vi "Planta lazo abierto.vi"() -> ()   [LabVIEW 2022 SP3]
uses:
  <vilib>/MakerHub/LINX/Public/Peripherals/PWM/PWM Set Duty Cycle 1 Chan.vi
  <vilib>/MakerHub/LINX/Public/Utilities/Open Serial.vi
  <vilib>/MakerHub/LINX/Public/Peripherals/PWM/PWM Set Duty Cycle N Chans.vi
  <vilib>/MakerHub/LINX/LMH-LINX.lvlib
panel:
  in  "Stop Button":bool
  out "Waveform Chart":cluster{dbl, dbl}(graph)
  in  "Set Point":dbl(slide) scale=0.0..100.0
  out "RPM":dbl(knob) scale=0.0..1500.0
  in  "Serial Port":refnum<visa-resource-name>="N/A"
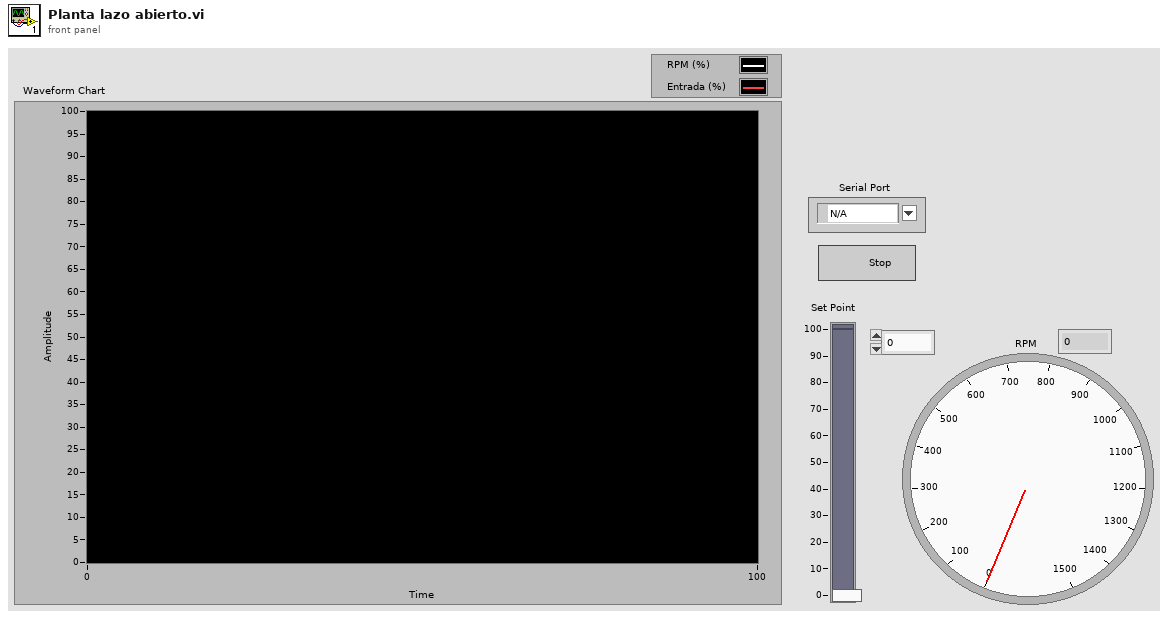
[diagram p1: front panel]
types:
  T1 = typedef "LMH-LINX.lvlib/LINX Ref.ctl" = cluster{"IO":T2, "Interface":T3, "LINX Device Config":T4}
  T2 = typedef "LMH-LINX.lvlib/Platform.ctl" = enum16{"Remote", "Local"}
  T3 = typedef "LMH-LINX.lvlib/Interface.ctl" = enum16{"Serial", "TCP"}
  T4 = typedef "LMH-LINX.lvlib/Device.lvlib/LINX Device Config.ctl" = cluster{"Interface":T3, "COM Port":refnum<visa-resource-name>, "TCP Configuration":T5, "Device Family":u8, "Device ID":u8, "Device Name":string, "TCP Ref":refnum<k5>, "Channels":T6}
  T5 = typedef "LMH-LINX.lvlib/Device.lvlib/TCP Config.ctl" = cluster{"IP Address":string, "Port":u16}
  T6 = typedef "LMH-LINX.lvlib/Channels.ctl" = cluster{"DI":u8[], "DO":u8[], "AI":u8[], "AO":u8[], "PWM":u8[], "QE":u8[], "UART":u8[], "I2C 2":u8[], "SPI":u8[], "CAN":u8[], "Servo":u8[], "AI Ref (V)":dbl, "AI Resolution (Bits)":u8, "AO Ref (V)":dbl, "AO Resolution (Bits)":u8}
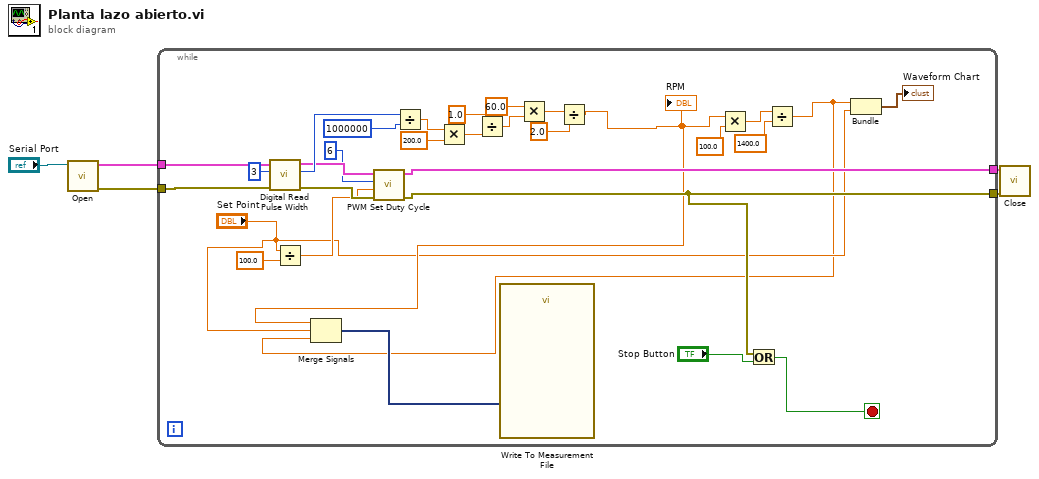
[diagram p0: block diagram]
diagram:
  n1 = call-poly <vilib>:"Open.vi"("Serial Port"="Serial Port") -> ("Error Out"=w3:errorcluster, "LINX Resource"=w4:T1)  [unwired: 8 in, 1 out]
  n2 = while {
    tunnel: w4 -> [w35]
    tunnel: w3 -> [w33]
    tunnel: [w24] -> w2
    tunnel: [w15] -> w1
    stop <- w17 stop-if-true
    n3 = call <vilib>:"Digital Read Pulse Width.vi"("Error In"=w33, "DI Channel"=u8 3, "LINX Resource"=w35) -> ("Error Out"=w23:errorcluster, "Pulse Width (uS)"=w32:u32, "LINX Resource"=w25:T1)  [unwired: 6 in]
    n4 = Divide(x="Set Point", y=100.0) -> (x/y=w9:dbl)
    n5 = call-poly <vilib>:"PWM Set Duty Cycle.vi"("Error In"=w23, "Duty Cycle (0-1)"=w9, "PWM Channel"=u8 6 ("DO Channel"), "LINX Resource"=w25) -> ("Error Out"=w15:errorcluster, "LINX Resource"=w24:T1)  [unwired: 6 in]
    n6 = Divide(x=w32, y=u32 1000000) -> (x/y=w30:dbl)
    n7 = Multiply(x=w30, y=200.0) -> (x*y=w28:dbl)
    n8 = Divide(x=1.0, y=w28) -> (x/y=w21:dbl)
    n9 = Multiply(x=60.0, y=w21) -> (x*y=w14:dbl)
    n10 = Divide(x=w14, y=2.0) -> (x/y=w10:dbl)
    "RPM" <- w10
    n11 = Multiply(x=w10, y=100.0) -> (x*y=w19:dbl)
    n12 = Or(x=w15, y="Stop Button") -> (x .or. y?=w17:bool)
    n13 = Divide(x=w19, y=1400.0) -> (x/y=w6:dbl)
    n14 = Merge Signals(w10, "Set Point", w6) -> (w11:dynamicdata)
    n15 = call "Write To Measurement File"("Signals"=w11) -> ()  [unwired: 16 in, 3 out]
    n16 = Bundle(w6, "Set Point"="Set Point") -> (→"Waveform Chart":cluster{dbl, "Set Point":dbl})  [unwired: 1 in]
  }
  n17 = call <vilib>:"Close.vi"("Error In"=w1, "LINX Resource"=w2) -> ()  [unwired: 9 in, 1 out]
